vi "FGMODE.vi"(1 "Mode":string, 2 "FG GPIB":i16=1) -> ()   [LabVIEW 2012]
panel:
  # "FGMD<space>[mode]"
  # "Mode list:\n\nM4: E.WID\nM1W3: Normal mode, square\nM1W4: Normal mode, pulse"
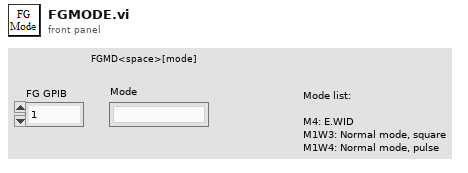
[diagram p1: front panel]
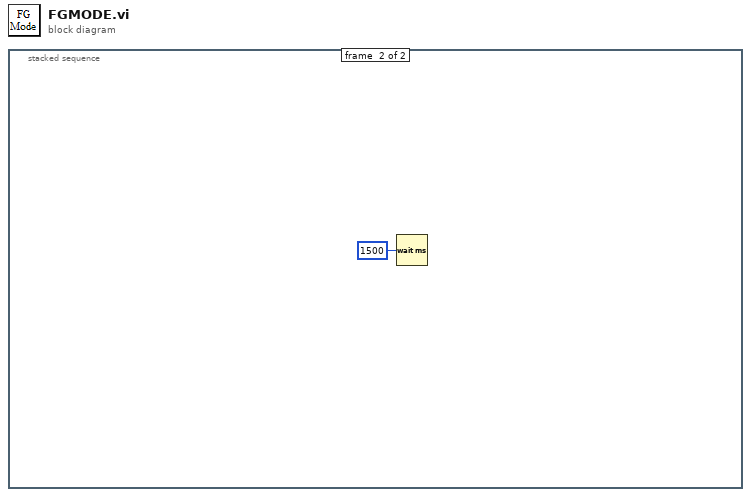
[diagram p0: block diagram]
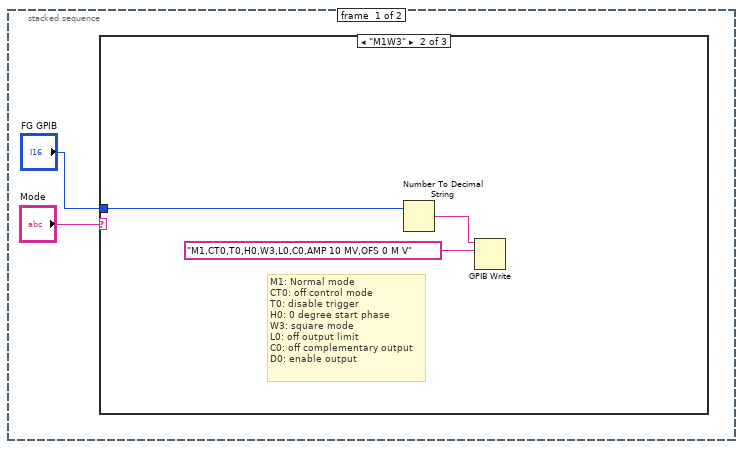
[diagram p2: hidden frame]
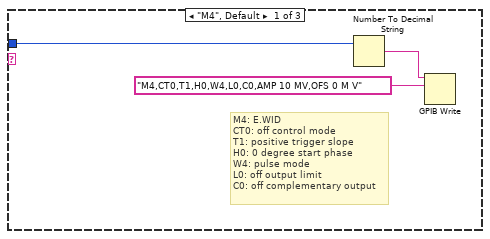
[diagram p3: hidden frame]
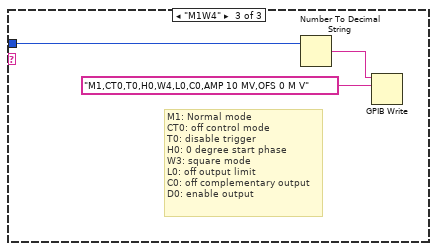
[diagram p4: hidden frame]
diagram:
  n1 = stacked-sequence {
    frame #0 {
      n2 = case shown="\"M1W3\"" "Mode" {
        tunnel: "FG GPIB" -> [w3 w7 w9]
        frame "M4", Default {
          # "M4: E.WID\nCT0: off control mode\nT1: positive trigger slope\nH0: 0 degree start phase\nW4: pulse mode\nL0: off output limit\nC0: off complementary output"
          n3 = Number To Decimal String(number=w3) -> (decimal integer string=w4:string)  [unwired: 1 in]
          n4 = GPIB Write(0:w4, 1:"M4,CT0,T1,H0,W4,L0,C0,AMP 10 MV,OFS 0 M V") -> ()  [unwired: 3 in, 2 out]
        }
        frame "M1W3" {
          # "M1: Normal mode\nCT0: off control mode\nT0: disable trigger\nH0: 0 degree start phase\nW3: square mode\nL0: off output limit\nC0: off complementary output\nD0: enable output"
          n5 = Number To Decimal String(number=w7) -> (decimal integer string=w8:string)  [unwired: 1 in]
          n6 = GPIB Write(0:w8, 1:"M1,CT0,T0,H0,W3,L0,C0,AMP 10 MV,OFS 0 M V") -> ()  [unwired: 3 in, 2 out]
        }
        frame "M1W4" {
          # "M1: Normal mode\nCT0: off control mode\nT0: disable trigger\nH0: 0 degree start phase\nW3: square mode\nL0: off output limit\nC0: off complementary output\nD0: enable output"
          n7 = Number To Decimal String(number=w9) -> (decimal integer string=w11:string)  [unwired: 1 in]
          n8 = GPIB Write(0:w11, 1:"M1,CT0,T0,H0,W4,L0,C0,AMP 10 MV,OFS 0 M V") -> ()  [unwired: 3 in, 2 out]
        }
      }
    }
    frame #1 {
      n9 = Wait (ms)(milliseconds to wait=u32 1500) -> ()  [unwired: 1 out]
    }
  }
